vi "WLAN - niVST - RFSA - Frequency and Level Settings.vi"(0 "instrument handle":refnum<k15>, 5 "TV Parameters(DataType)":T2 {"Standard" items=["80211A/G/J/P OFDM", "80211B/G DSSS", "80211G DSSSOFDM", "80211N MIMOOFDM", "80211AC MIMOOFDM"]; "OFDM Data Rate (Mbps)" items=["6", "9", "12", "18", "24", "36", "48", "54"]; "80211n PLCP Frame Format" items=["Mixed Format", "Greenfield Format"]; "FEC Coding Type" items=["BCC", "LDPC"]; "DSSS Data Rate (Mbps)" items=["1", "2", "5.5 CCK", "5.5 PBCC", "11 CCK", "11 PBCC", "22", "33"]}, 7 "PL":T1, 11 "error in":errorcluster) -> (4 "instrument handle":refnum<k15>, 15 "error out":errorcluster)   [LabVIEW 2012]
uses:
  TV/RW/Includes/WLAN - TV - RW - INC - TV_DataType_Cluster.ctl
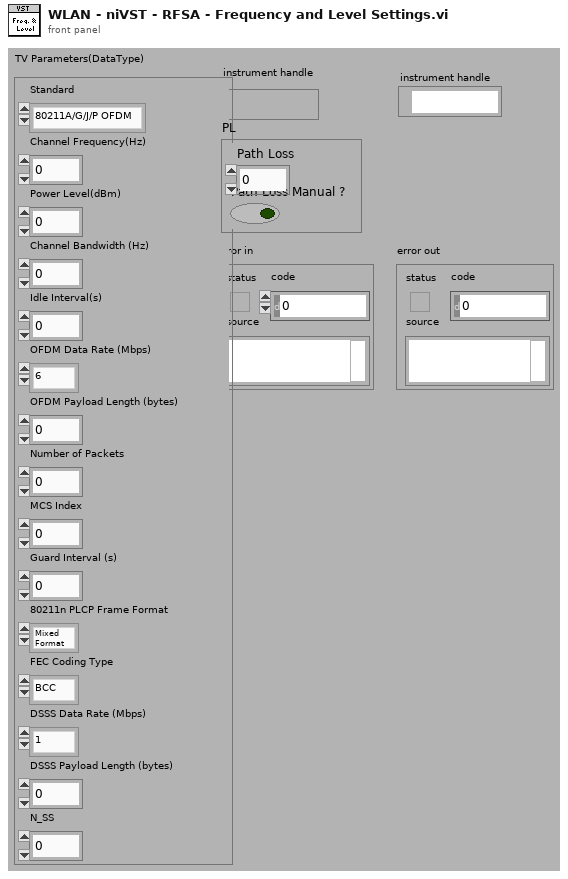
[diagram p1: front panel]
types:
  T1 = cluster{"Path Loss":dbl, "Path Loss Manual ?":bool}
  T2 = typedef "WLAN - TV - RW - INC - TV_DataType_Cluster.ctl" = cluster{"Standard":i32, "Channel Frequency(Hz)":dbl, "Power Level(dBm)":dbl, "Channel Bandwidth (Hz)":dbl, "Idle Interval(s)":dbl, "OFDM Data Rate (Mbps)":i32, "OFDM Payload Length (bytes)":i32, "Number of Packets":i32, "MCS Index":i32, "Guard Interval (s)":dbl, "80211n PLCP Frame Format":i32, "FEC Coding Type":i32, "DSSS Data Rate (Mbps)":i32, "DSSS Payload Length (bytes)":i32, "N_SS":i32}
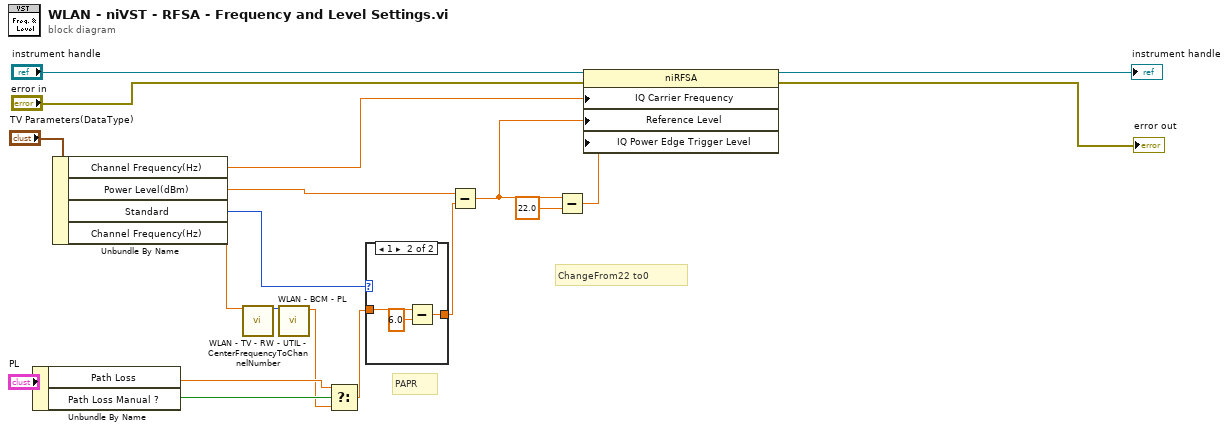
[diagram p0: block diagram]
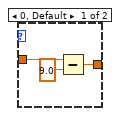
[diagram p2: hidden frame]
diagram:
  # "ChangeFrom22 to0"
  # "PAPR"
  n1 = Unbundle By Name("PL") -> ("Path Loss"=w3:dbl, "Path Loss Manual ?"=w4:bool)
  n2 = Unbundle By Name("TV Parameters(DataType)") -> ("Channel Frequency(Hz)"=w12:dbl, "Power Level(dBm)"=w11:dbl, "Standard"=w9:i32, "Channel Frequency(Hz)"=w8:dbl)
  n3 = call "WLAN - TV - RW - UTIL - CenterFrequencyToChannelNumber.vi"("Center Frequency(Hz)"=w8) -> ("Coherced Channel Number"=w5:i32)  [unwired: 13 in, 1 out]
  n4 = call "WLAN - BCM - PL.vi"("Channel index"=w5) -> ("PL"=w1:dbl)  [unwired: 10 in]
  n5 = Select(t=w3, s=w4, f=w1) -> (s? t:f=w2:dbl)
  n6 = case shown="1" w9 {
    tunnel: w2 -> [w22 w24]
    tunnel: [w20 w23] -> w7
    frame 0, Default {
      n7 = Subtract(x=w22, y=9.0) -> (x-y=w20:dbl)
    }
    frame 1 {
      n8 = Subtract(x=w24, y=6.0) -> (x-y=w23:dbl)
    }
  }
  n9 = Subtract(x=w11, y=w7) -> (x-y=w10:dbl)
  n10 = Subtract(x=w10, y=22.0) -> (x-y=w18:dbl)
  n11 = property class="niRFSA"(reference="instrument handle", error in="error in", "IQ Carrier Frequency"=w12, "Reference Level"=w10, "IQ Power Edge Trigger Level"=w18) -> (reference out=→"instrument handle":refnum<k15>, error out=→"error out":errorcluster)
